vi "toml_loads.vi"(8 "error in (no error)":errorcluster, 11 "toml":string) -> (0 "error out":errorcluster, 3 "variant":variant)   [LabVIEW 2017]
panel:
  # "'a':{\n'b':{\n'c':{\n    'a':{'b':40}\n}\n}\n}"
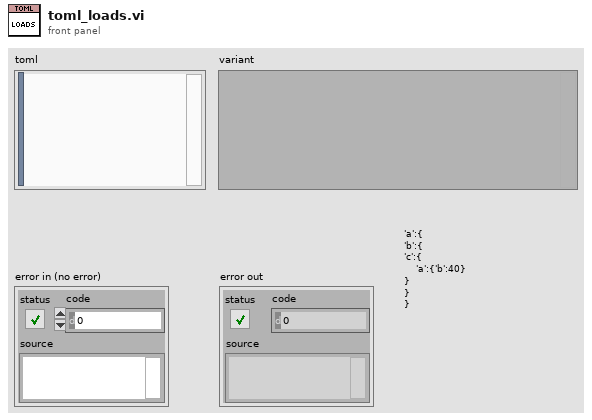
[diagram p1: front panel]
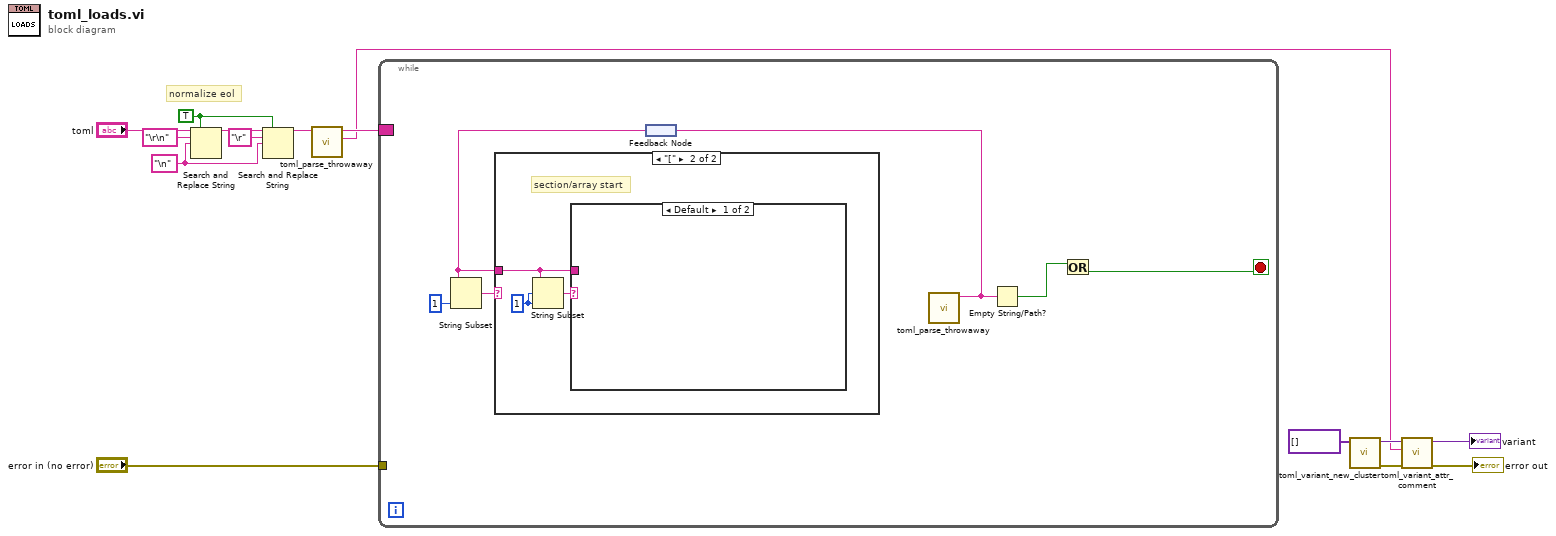
[diagram p0: block diagram]
diagram:
  w13 = "\n" ("search string")
  w12 = TRUE ("replace all? (F)")
  # "normalize eol"
  n1 = Search and Replace String(replace all?=w12, input string="toml", search string="\r\n", replace string=w13) -> (result string=w10:string)  [unwired: 4 in, 3 out]
  n2 = Search and Replace String(replace all?=w12, input string=w10, search string="\r", replace string=w13) -> (result string=w8:string)  [unwired: 4 in, 3 out]
  n3 = call "toml_parse_throwaway.vi"("string in"=w8) -> ("comments"=w2:string, "string out"=w7:string)  [unwired: 9 in]
  n4 = while {
    tunnel: "error in (no error)" -> [_]
    border: w7 -> [_]
    stop <- w21 stop-if-true
    n5 = feedback #1() -> (w16:string)
    n6 = String Subset(string=w16, length (rest)=1 ("length (rest)")) -> (substring=w17:string)  [unwired: 1 in]
    n7 = case shown="\"[\"" w17 {
      tunnel: w16 -> [_ w22]
      frame "False", Default {
      }
      frame "[" {
        w24 = 1 ("length (rest)")
        # "section/array start"
        n8 = String Subset(string=w22, offset (0)=w24, length (rest)=w24) -> (substring=w23:string)
        n9 = case shown="Default" w23 {
          tunnel: w22 -> [_ _]
          frame Default {
          }
          frame "[" {
          }
        }
      }
    }
    n10 = call "toml_parse_throwaway.vi"() -> ("string out"=w20:string)  [unwired: 10 in, 1 out]
    n11 = feedback-in #1(w20) -> ()
    n12 = Empty String/Path?(string/path=w20) -> (empty?=w19:bool)
    n13 = Or(x=w19) -> (x .or. y?=w21:bool)  [unwired: 1 in]
  }
  n14 = call "toml_variant_new_cluster.vi"("elements"=variant[] []) -> ("error out"=w6:errorcluster, "cluster"=w4:variant)  [unwired: 9 in]
  n15 = call "toml_variant_attr_comment.vi"("error in (no error)"=w6, "comment"=w2, "variant in"=w4) -> ("error out"=→"error out":errorcluster, "variant out"=→"variant":variant)  [unwired: 7 in]
